vi "background launcher.vi"(9 "comm return queue":refnum<queue>, 10 "queue size (1,10000)":i32=1000, 11 "communicator in":refnum<class "communicator.lvclass">) -> ()   [LabVIEW 2015]
uses:
  communicator.lvclass
  communicator queue/identifying queue.lvclass
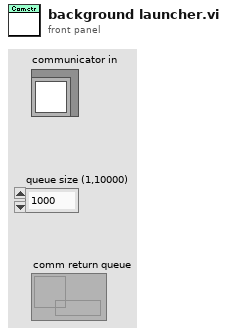
[diagram p1: front panel]
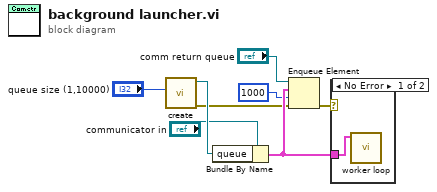
[diagram p0: block diagram]
diagram:
  n1 = call "create.vi"("size (1,10000)"="queue size (1,10000)") -> ("error out"=w2:errorcluster, "message connection out"=w8:refnum<class "identifying queue.lvclass">)  [unwired: 9 in]
  n2 = Bundle By Name(cluster="communicator in", "queue"=w8) -> (w4:cluster{})
  n3 = Enqueue Element(queue="comm return queue", element=w4, timeout in ms (-1)=1000, error in (no error)=w2) -> (error out=w1:errorcluster)  [unwired: 2 out]
  n4 = case shown="No Error" w1 {
    tunnel: w4 -> [w9 _]
    frame No Error {
      n5 = call "worker loop.vi"("communicator in"=w9) -> ()  [unwired: 11 in]
    }
    frame Error {
    }
  }
